vi "PLC.WriteToFile.vi"(7 "Idx":i32, 8 "error in":errorcluster, 10 "Data":T1 {"Values" format="%.3f"}) -> (0 "error out":errorcluster, 1 "Data saved":bool)   [LabVIEW 2016]
doc: "Write test results (measurement values) to proda database\n\nWabco 2017 All right reserved\nAuthor: maciej.szupienko@wabco-auto.com"
uses:
  Subvis/StepStatus.ctl
  LowLevel/PLC.DataBlock.PLCvalues.ctl
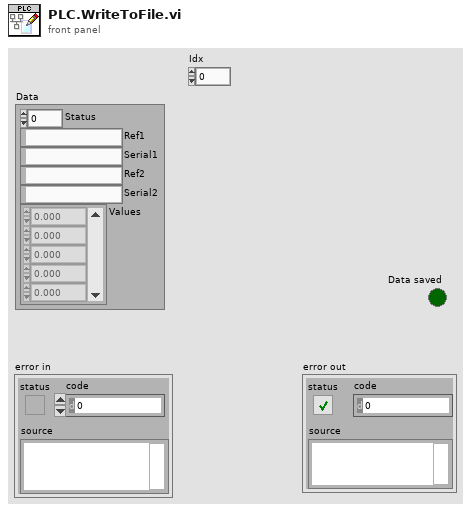
[diagram p1: front panel]
types:
  T1 = typedef "PLC.DataBlock.PLCvalues.ctl" = cluster{"Status":u8, "Ref1":string, "Serial1":string, "Ref2":string, "Serial2":string, "Values":sgl[]}
  T2 = typedef "StepStatus.ctl" = enum16{"-", "Pending", "Running", "Skipped", "Passed", "Failed", "Done", "Error", "Aborted", "Stopped"}
  T3 = typedef "Cache.TestSteps.Fglb.ResultData.ctl" = cluster{"Ref":string, "Serial":string, "Pr":T4, "PSr":T5, "TSr":cluster{"TSr":T6, "TVr":T7[]}[]}
  T4 = typedef "ProdaNG.ProcessResult.ctl" = cluster{"c_id":string, "productId":string, "processId":i32, "statusId":i32, "startTime":string, "endTime":string}
  T5 = typedef "ProdaNG.ProcessStepResult.ctl" = cluster{"c_id":string, "processResultId":string, "processStepId":i32, "statusId":i32, "operatorId":i32, "startTime":string, "endTime":string}
  T6 = typedef "ProdaNG.TestStepResult.ctl" = cluster{"c_id":string, "processStepResultId":string, "testStepId":i32, "statusId":i32}
  T7 = typedef "ProdaNG.TestValueResult.ctl" = cluster{"c_id":string, "testStepResultId":string, "testValueId":i32, "result":dbl, "statusId":i32, "contentId":string}
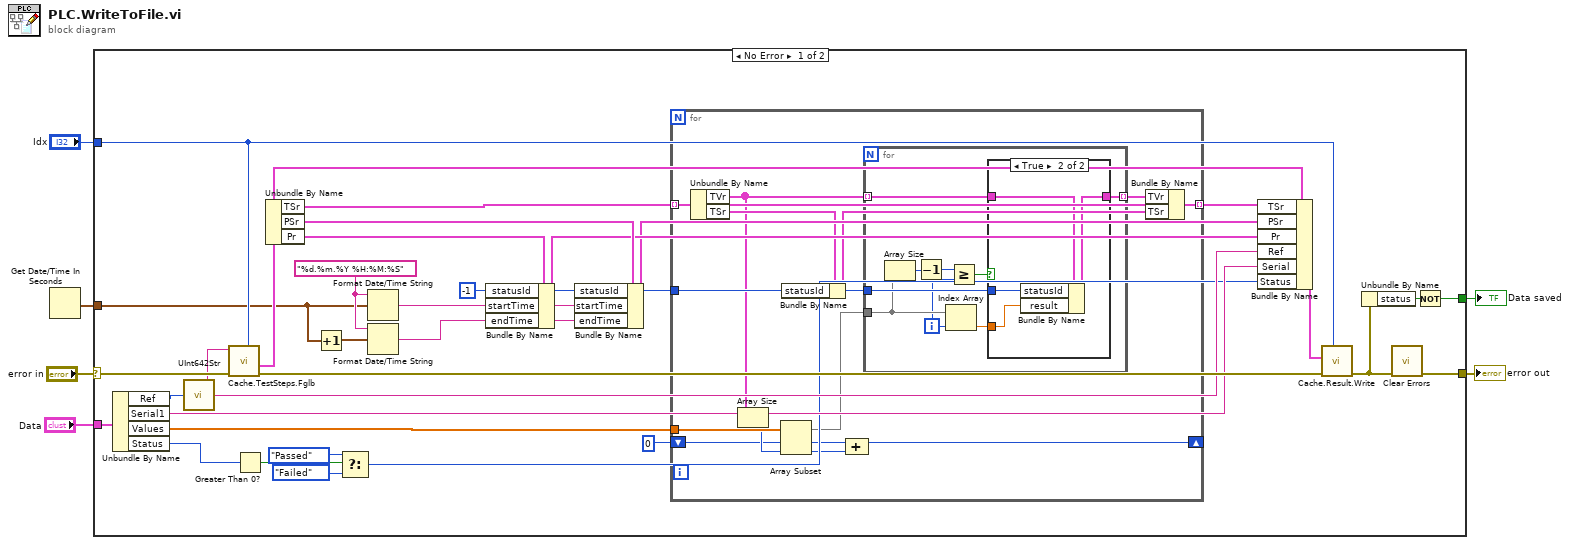
[diagram p0: block diagram]
diagram:
  n1 = Get Date/Time In Seconds() -> (seconds since 1Jan1904=w2:timestamp)
  n2 = case shown="No Error" "error in" {
    selector: "error in" -> [w38 w65]
    tunnel: [w18 w65] -> w6
    tunnel: "Data" -> [w37 _]
    tunnel: "Idx" -> [w19 _]
    tunnel: [w15 _] -> w3
    tunnel: w2 -> [w14 _]
    frame No Error {
      w31 = "%d.%m.%Y %H:%M:%S" ("time format string (%c)")
      w29 = -1 ("statusId")
      n3 = Unbundle By Name(w37) -> ("Ref"=w10:u64, "Serial1"=w20:string, "Values"=w36:sgl[], "Status"=w8:u8)
      n4 = call "UInt642Str.vi"("Numeric"=w10) -> ("string"=w9:string)
      n5 = call "Cache.TestSteps.Fglb.vi"("SystemIdx"=w19, "error in (no error)"=w38, "Variant"=w9) -> ("error out"=w22:errorcluster, "Result out"=w26:T3)  [unwired: 5 in, 2 out]
      n6 = Greater Than 0?(x=w8) -> (x > 0?=w13:bool)
      n7 = Unbundle By Name(w26) -> ("TSr"=w35:cluster{"TSr":T6, "TVr":T7[]}[], "PSr"=w34:T5, "Pr"=w33:T4)
      n8 = Increment(x=w14) -> (x+1=w30:timestamp)
      n9 = Select(t=StepStatus."Passed" ("StepStatus"), s=w13, f=StepStatus."Failed" ("StepStatus")) -> (s? t:f=w7:T2)
      n10 = Format Date/Time String(time format string (%c)=w31, seconds (now)=w14) -> (date/time string=w28:string)  [unwired: 1 in]
      n11 = Format Date/Time String(time format string (%c)=w31, seconds (now)=w30) -> (date/time string=w27:string)  [unwired: 1 in]
      n12 = Bundle By Name(cluster=w33, "statusId"=w29, "startTime"=w28, "endTime"=w27) -> (w24:T4)
      n13 = Bundle By Name(cluster=w34, "statusId"=w29, "startTime"=w28, "endTime"=w27) -> (w23:T5)
      n14 = for {
        tunnel: w36 -> [w45]
        tunnel: w35 -> [w49] mode=indexing
        tunnel: w29 -> [w50]
        tunnel: [w46] -> w25 mode=indexing
        shift-right: [w40] -> _
        shift-left: 0 -> [w42]
        n15 = Unbundle By Name(w49) -> ("TVr"=w44:T7[], "TSr"=w47:T6)
        n16 = Array Size(array=w44) -> (size(s)=w43:i32)
        n17 = Array Subset(array=w45, index=w42, length=w43) -> (w41:sgl[])
        n18 = Bundle By Name(cluster=w47, "statusId"=w50) -> (w39:T6)
        n19 = Compound Arithmetic op=ADD(w42, w43) -> (w40:i32)
        n20 = for "results" {
          tunnel: w41 -> [w55]
          tunnel: w50 -> [w59]
          tunnel: w44 -> [w58] mode=indexing
          tunnel: [w57] -> w48 mode=indexing
          i -> [w53]
          n21 = Array Size(array=w55) -> (size(s)=w52:i32)
          n22 = Decrement(x=w52) -> (x-1=w51:i32)
          n23 = Index Array(array=w55, index=w53) -> (element=w56:sgl)
          n24 = Greater Or Equal?(x=w51, y=w53) -> (x >= y?=w54:bool)
          n25 = case shown="True" w54 {
            tunnel: w59 -> [_ w64]
            tunnel: w58 -> [w60 w63]
            tunnel: [w60 w62] -> w57
            tunnel: w56 -> [_ w61]
            frame False {
            }
            frame True {
              n26 = Bundle By Name(cluster=w63, "statusId"=w64, "result"=w61) -> (w62:T7)
            }
          }
        }
        n27 = Bundle By Name(cluster=w49, "TVr"=w48, "TSr"=w39) -> (w46:cluster{"TSr":T6, "TVr":T7[]})
      }
      n28 = Bundle By Name(cluster=w26, "TSr"=w25, "PSr"=w23, "Pr"=w24, "Ref"=w9, "Serial"=w20, "Status"=w7) -> (w21:T3)
      n29 = call "Cache.Result.Write.vi"("Station"=w19, "error in (no error)"=w22, "Result in"=w21) -> ("error out"=w17:errorcluster)  [unwired: 8 in]
      n30 = Unbundle By Name(w17) -> ("status"=w16:bool)
      n31 = call <vilib>:"Clear Errors.vi"("error in (no error)"=w17) -> ("error out"=w18:errorcluster)  [unwired: 5 in, 1 out]
      n32 = Not(x=w16) -> (.not. x?=w15:bool)
    }
    frame Error {
    }
  }
  "error out" <- w6
  "Data saved" <- w3
